vi "Get_TCPrefnum.vi"(8 "error in":errorcluster) -> (0 "error out":errorcluster, 3 "Socket out":refnum<class "Socket.lvclass">)   [LabVIEW 2020]
uses:
  WebSockets-API/Source/Sockets/Socket/Socket.lvclass
  WebSockets-API/Source/Sockets/VISA TCP Listener/VISA TCP Listener.lvclass
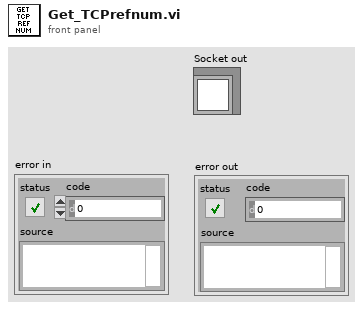
[diagram p1: front panel]
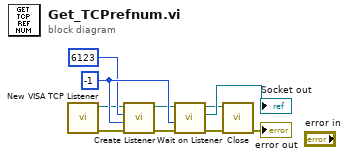
[diagram p0: block diagram]
diagram:
  w8 = -1 ("timeout ms (25000)")
  n1 = call "New VISA TCP Listener.vi"() -> ("error out"=w2:errorcluster, "VISA TCP Listener out"=w1:refnum<class "VISA TCP Listener.lvclass">)  [unwired: 10 in]
  n2 = call-dynamic "Create Listener.vi"("error in (no error)"=w2, "timeout ms (5000)"=w8, "Port"=u16 6123 ("port"), "VISA TCP Listener in"=w1) -> ("error out"=w4:errorcluster, "VISA TCP Listener out"=w6:refnum<class "VISA TCP Listener.lvclass">)  [unwired: 6 in]
  n3 = call-dynamic "Wait on Listener.vi"("error in (no error)"=w4, "timeout ms (5000)"=w8, "VISA TCP Listener in"=w6) -> ("error out"=w3:errorcluster, "Socket out"=→"Socket out":refnum<class "Socket.lvclass">, "VISA TCP Listener out"=w5:refnum<class "VISA TCP Listener.lvclass">)  [unwired: 6 in]
  n4 = call-dynamic "Close.vi"("error in (no error)"=w3, "VISA TCP Listener in"=w5) -> ("error out"=→"error out":errorcluster)  [unwired: 9 in]
